vi "ITC503-RunRampT.vi"(1 "Rate (K/min)":dbl format="%#_13g", 2 "Final T (K)":dbl format="%#_13g") -> ()   [LabVIEW 2019]
uses:
  Global/Global Variables/Data_Display_global.vi
  Instrument_Setup.vi
panel:
  out "K/s":dbl format="%#_13g"
  out "Current Setpoint":dbl format="%#_13g"
  out "Sweep Time":dbl format="%#_13g"
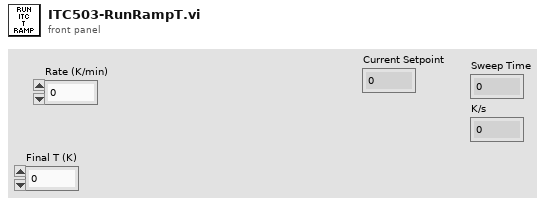
[diagram p1: front panel]
types:
  T1 = typedef "ITC503Monitor-Cluster.ctl" = cluster{"Temperatur (K)":dbl, "Setpoint (K)":dbl, "Rate (K/min)":dbl, "Heater (%)":dbl, "NV (%)":dbl, "Heater Manual":bool, "NV Manual":bool, "Go to Set":bool, "Heater SP":dbl, "Valid?":bool, "Set Heater SP":bool, "Set NV SP":bool, "Heater (%) Display":dbl, "NV (%) Display":dbl, "NV Setpoint":dbl, "Change Heater Status":bool, "Change NV Status":bool, "Sample 3":dbl, "Sample 2":dbl, "Sweep-State":bool, "Set Auto PID":bool, "Auto PID":bool, "Stopp":bool, "Setpoint-Sweep":dbl, "Sample 1":dbl, "Control Channel":bool, "Channel 1":bool, "Channel 2":bool, "Channel 3":bool}
  T2 = cluster{"Com Port":i32, "ISOBUS Address":i32, "GPIB Address":i16, "Communication":enum16{"RS232", "ISOBUS", "GPIB", "Gateway"}}
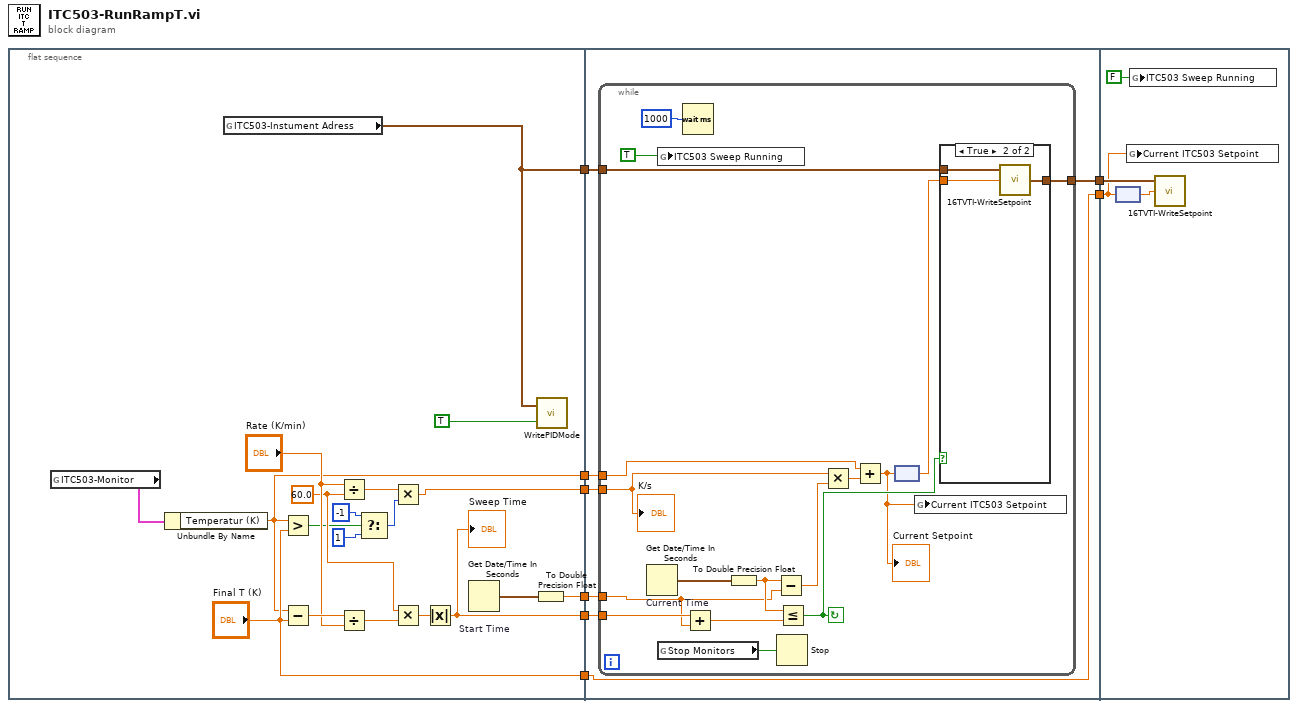
[diagram p0: block diagram]
diagram:
  n1 = flat-sequence {
    tunnel: [w11] -> w8
    tunnel: [w16] -> w7
    tunnel: [w24] -> w6
    tunnel: [w19] -> w5
    tunnel: ["Final T (K)"] -> w4
    tunnel: [w9] -> w3
    tunnel: w8 -> [w34]
    tunnel: w7 -> [w33]
    tunnel: w6 -> [w32]
    tunnel: w5 -> [w31]
    tunnel: [w30] -> w2
    tunnel: w4 -> [w30]
    tunnel: w3 -> [w29]
    tunnel: [w28] -> w1
    tunnel: w2 -> [w57]
    tunnel: w1 -> [w58]
    frame #0 {
      w21 = 60.0
      n2 = global read "Data_Display_global.vi" "ITC503-Monitor"() -> (w27:T1)
      n3 = Unbundle By Name(w27) -> ("Temperatur (K)"=w16:dbl)
      n4 = global read "Instrument_Setup.vi" "ITC503-Instument Adress"() -> (w9:T2)
      n5 = Greater?(x=w16, y="Final T (K)") -> (0:w15:bool)
      n6 = Subtract(x=w16, y="Final T (K)") -> (x-y=w26:dbl)
      n7 = Divide(x="Rate (K/min)", y=w21) -> (x/y=w12:dbl)
      n8 = Divide(x=w26, y="Rate (K/min)") -> (x/y=w22:dbl)
      n9 = Select(t=-1, s=w15, f=1) -> (s? t:f=w10:i32)
      n10 = Multiply(x=w12, y=w10) -> (x*y=w11:dbl)
      n11 = Multiply(x=w21, y=w22) -> (x*y=w20:dbl)
      n12 = Absolute Value(x=w20) -> (abs(x)=w19:dbl)
      "Sweep Time" <- w19
      n13 = Get Date/Time In Seconds "Start Time"() -> (seconds since 1Jan1904=w25:timestamp)
      n14 = To Double Precision Float(number=w25) -> (double precision float=w24:dbl)
      n15 = call "WritePIDMode.vi"("Auto PID"=TRUE, "Instrument address"=w9) -> ()  [unwired: 1 in, 1 out]
    }
    frame #1 {
      n16 = while {
        tunnel: w34 -> [w49]
        tunnel: w33 -> [w46]
        tunnel: w32 -> [w39]
        tunnel: w31 -> [w45]
        tunnel: w29 -> [w42]
        tunnel: [w41] -> w28
        stop <- w38 continue-if-true
        n17 = Get Date/Time In Seconds "Current Time"() -> (seconds since 1Jan1904=w51:timestamp)
        n18 = global write "Data_Display_global.vi" "ITC503 Sweep Running"(TRUE) -> ()
        n19 = global read "Data_Display_global.vi" "Stop Monitors"() -> (w35:bool)
        n20 = Wait (ms)(milliseconds to wait=1000) -> ()  [unwired: 1 out]
        n21 = Add(x=w45, y=w39) -> (x+y=w44:dbl)
        n22 = To Double Precision Float(number=w51) -> (double precision float=w40:dbl)
        n23 = Subtract(x=w40, y=w39) -> (x-y=w50:dbl)
        n24 = Stop(stop? (T)=w35) -> ()
        n25 = Less Or Equal?(x=w40, y=w44) -> (x <= y?=w38:bool)
        n26 = Multiply(x=w49, y=w50) -> (x*y=w48:dbl)
        n27 = Add(x=w46, y=w48) -> (x+y=w37:dbl)
        "Current Setpoint" <- w37
        n28 = node(w37) -> (w43:dbl[unit])
        n29 = global write "Data_Display_global.vi" "Current ITC503 Setpoint"(w37) -> ()
        n30 = case shown="True" w38 {
          tunnel: w43 -> [_ w55]
          tunnel: w42 -> [w52 w54]
          tunnel: [w52 w53] -> w41
          frame False {
          }
          frame True {
            n31 = call "16TVTI-WriteSetpoint.vi"("Set point"=w55, "Instrument address"=w54) -> ("Instrument address (out)"=w53:T2)  [unwired: 1 in]
          }
        }
        "K/s" <- w49
      }
    }
    frame #2 {
      n32 = node(w57) -> (w59:dbl[unit])
      n33 = global write "Data_Display_global.vi" "Current ITC503 Setpoint"(w57) -> ()
      n34 = global write "Data_Display_global.vi" "ITC503 Sweep Running"(FALSE) -> ()
      n35 = call "16TVTI-WriteSetpoint.vi"("Set point"=w59, "Instrument address"=w58) -> ()  [unwired: 1 in, 1 out]
    }
  }
